vi "Receive.vi"(8 "error in (no error)":errorcluster, 11 "Tovey9150 in":refnum<class "Tovey 9150.lvclass">) -> (0 "error out":errorcluster, 2 "Response":string, 3 "Tovey9150 out":refnum<class "Tovey 9150.lvclass">)   [LabVIEW 2015, in "Tovey 9150.lvclass"]
uses:
  Tovey 9150.lvclass
  Tovey 9150.lvclass/Tovey 9150.ctl
  Common_SerialProtocols/SerialCommunicator/SerialCommunicator.lvclass
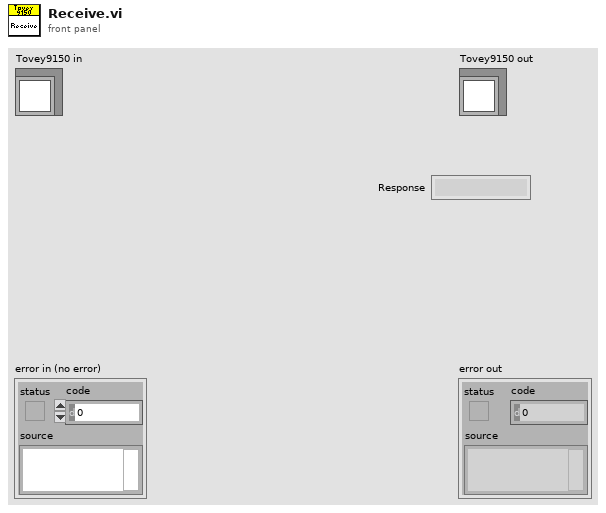
[diagram p1: front panel]
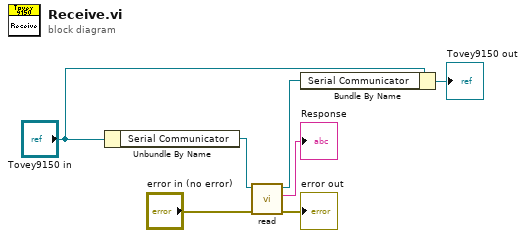
[diagram p0: block diagram]
diagram:
  n1 = Unbundle By Name("Tovey9150 in") -> ("Serial Communicator"=w5:refnum<class "SerialCommunicator.lvclass">)
  n2 = call-dynamic "read.vi"("error in (no error)"="error in (no error)", "SerialCommunicator in"=w5) -> ("error out"=→"error out":errorcluster, "stringRead"=→"Response":string, "SerialCommunicator out"=w4:refnum<class "SerialCommunicator.lvclass">)  [unwired: 7 in]
  n3 = Bundle By Name(cluster="Tovey9150 in", "Serial Communicator"=w4) -> (→"Tovey9150 out":refnum<class "Tovey 9150.lvclass">)
